vi "Print PDF.vi"(7 "printSettings":refnum<k24>, 8 "Error In":errorcluster, 9 "Timeout ms":i32, 10 "PDF File Path":path, 11 "WebView in":refnum<class "WebView.lvclass">) -> (0 "Error Out":errorcluster, 2 "Timeout":bool, 3 "WebView out":refnum<class "WebView.lvclass">)   [LabVIEW 2024, in "WebView.lvclass"]
uses:
  WebView.lvclass
  WebView.lvclass/WebView.ctl
  <vilib>/sklein/WebView2/Libs/Microsoft.Web.WebView2.Core.dll
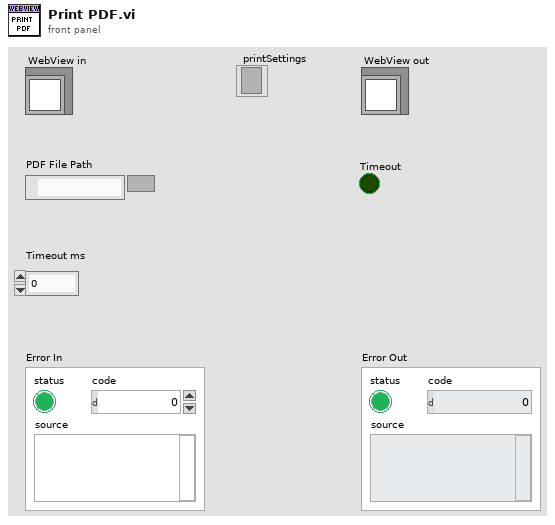
[diagram p1: front panel]
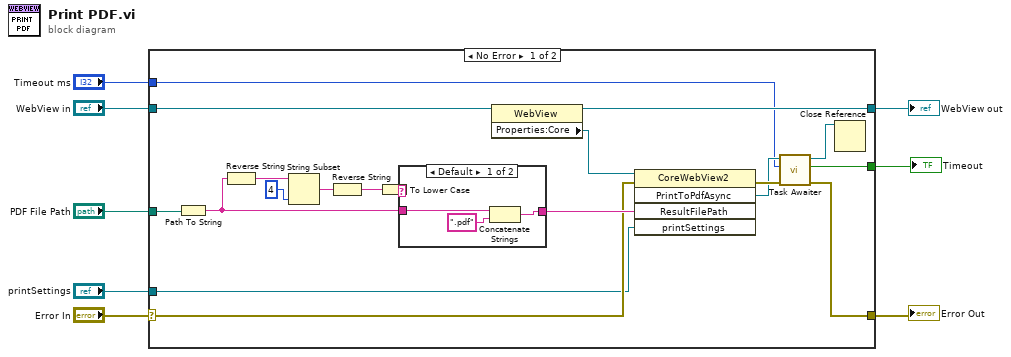
[diagram p0: block diagram]
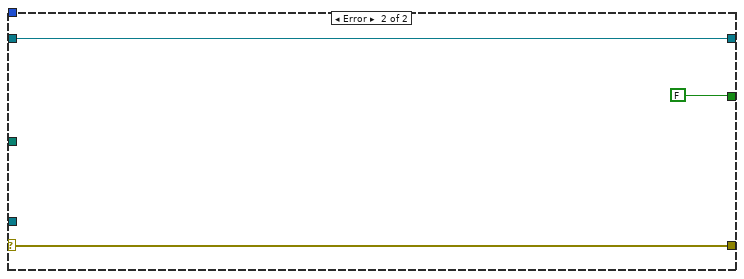
[diagram p3: hidden frame]
diagram:
  n1 = case shown="No Error" "Error In" {
    selector: "Error In" -> [w18 w34]
    tunnel: [w11 w34] -> w7
    tunnel: [w17 w33] -> w5
    tunnel: "WebView in" -> [w27 w33]
    tunnel: "PDF File Path" -> [w19 _]
    tunnel: [w12 FALSE ("Timeout")] -> w3
    tunnel: "Timeout ms" -> [w10 _]
    tunnel: "printSettings" -> [w9 _]
    frame No Error {
      n2 = Path To String(path=w19) -> (string=w20:string)
      n3 = Reverse String(1:w20) -> (0:w26:string)
      n4 = String Subset(string=w26, length (rest)=4 ("length (rest)")) -> (substring=w24:string)  [unwired: 1 in]
      n5 = Reverse String(1:w24) -> (0:w23:string)
      n6 = To Lower Case(string=w23) -> (all lower case string=w22:string)
      n7 = case shown="Default" w22 {
        tunnel: [w28 w31] -> w21
        tunnel: w20 -> [w30 w31]
        frame Default {
          n8 = Concatenate Strings(w30, ".pdf" ("string")) -> (w28:string)
        }
        frame ".pdf" {
        }
      }
      n9 = property class="WebView"(reference=w27) -> (reference out=w17:refnum<class "WebView.lvclass">, "Properties:Core"=w16:refnum<k24>)  [unwired: 1 in, 1 out]
      n10 = invoke class="CoreWebView2" method="PrintToPdfAsync"(reference=w16, error in=w18, "ResultFilePath"=w21, "printSettings"=w9) -> (error out=w15:errorcluster, "PrintToPdfAsync"=w14:refnum<k24>)  [unwired: 1 in, 3 out]
      n11 = call "Task Awaiter.vi"("error in (no error)"=w15, "Timeout"=w10, "Task"=w14) -> ("error out"=w11:errorcluster, "Timeout"=w12:bool, "Task"=w13:refnum<k24>)  [unwired: 6 in]
      n12 = Close Reference(reference=w13) -> ()  [unwired: 1 in, 1 out]
    }
    frame Error {
    }
  }
  "Error Out" <- w7
  "WebView out" <- w5
  "Timeout" <- w3
